vi "Find Available Cell.vi"(8 "error in (no error)":errorcluster, 10 "Indexes":cluster{"Row":i16, "Column":i16}, 11 "Board in":refnum<class "Board.lvclass">) -> (0 "error out":errorcluster, 1 "Free Cell Found":bool, 2 "Available Indexes":cluster{i32, i32}, 3 "Board out":refnum<class "Board.lvclass">)   [LabVIEW 2017, in "Board.lvclass"]
uses:
  Board.lvclass
  Board.lvclass/Board.ctl
  <vilib>/LIEF/Forms/Shape/Shape.lvclass
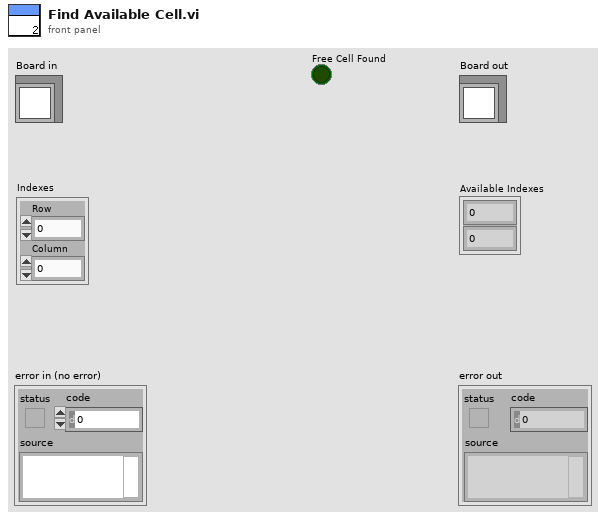
[diagram p1: front panel]
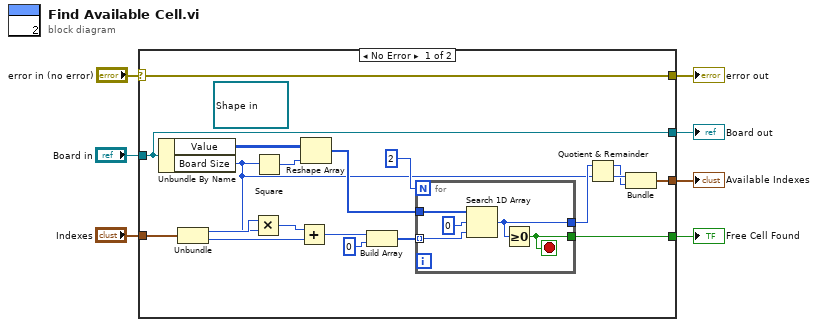
[diagram p0: block diagram]
diagram:
  n1 = case shown="No Error" "error in (no error)" {
    selector: "error in (no error)" -> [w26 w33]
    tunnel: [w26 w33] -> w6
    tunnel: [w24 w32] -> w4
    tunnel: "Board in" -> [w24 w32]
    tunnel: "Indexes" -> [w25 _]
    tunnel: [w15 _] -> w2
    tunnel: [w10 _] -> w1
    frame No Error {
      (unwired) refnum<data-value> refnum ("New Block")
      n2 = Unbundle By Name(w24) -> ("Value"=w23:u32[][], "Board Size"=w9:u16)
      n3 = Unbundle(w25) -> ("Row"=w21:i16, "Column"=w19:i16)
      n4 = Multiply(x=w21, y=w9) -> (x*y=w20:u16)
      n5 = Square(x=w9) -> (x^2=w8:u16)
      n6 = Add(x=w20, y=w19) -> (x+y=w14:u16)
      n7 = Reshape Array(w23, w8) -> (w22:u32[])
      n8 = Build Array(w14, u16 0 ("element")) -> (w12:u16[])
      n9 = for {
        N: 2 -> [_]
        tunnel: w22 -> [w31]
        tunnel: w12 -> [w30] mode=indexing
        tunnel: [w29] -> w18
        tunnel: [w28] -> w10
        stop <- w28 stop-if-true
        n10 = Search 1D Array(1D array=w31, element=u32 0, start index (0)=w30) -> (index of element=w29:i32)
        n11 = Greater Or Equal To 0?(x=w29) -> (x >= 0?=w28:bool)
      }
      n12 = Quotient & Remainder(x=w18, y=w9) -> (x-y*floor(x/y)=w16:i32, floor(x/y)=w17:i32)
      n13 = Bundle(w17, w16) -> (w15:cluster{i32, i32})  [unwired: 1 in]
    }
    frame Error {
    }
  }
  "error out" <- w6
  "Board out" <- w4
  "Available Indexes" <- w2
  "Free Cell Found" <- w1
